vi "Start.vi"(8 "error in":errorcluster, 9 "timeout (-1)":i32=-1, 11 "Standard Engine Runtime in":refnum<class "Standard Engine Runtime.lvclass">) -> (0 "error out":errorcluster, 3 "Standard Engine Runtime out":refnum<class "Standard Engine Runtime.lvclass">)   [LabVIEW 2013, in "Standard Engine Runtime.lvclass"]
doc: "Sends a command for a paused but initialized engine to begin execution and enter the 'Running' state."
uses:
  Standard Engine Runtime.lvclass
  <vilib>/NI/Module Execution Interface/Engine Runtime/Execution States.ctl
  Standard Engine Runtime.lvclass/Standard Engine Runtime.ctl
  <vilib>/NI/Module Execution Interface/Engine Runtime/Engine Runtime Interface.lvclass
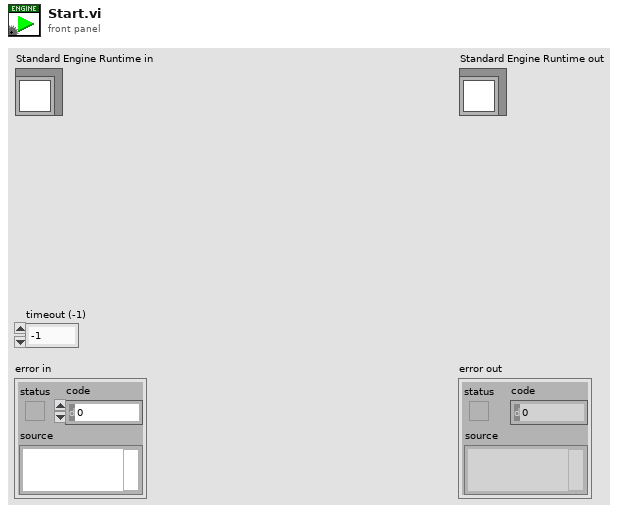
[diagram p1: front panel]
types:
  T1 = typedef "Engine Runtime Interface.lvclass/Execution States.ctl" = enum16{"Init", "Pre-Operational", "Safe-Operational", "Operational", "Stopped"}
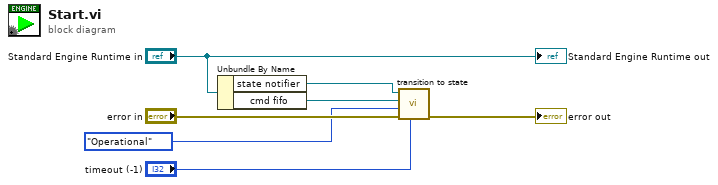
[diagram p0: block diagram]
diagram:
  n1 = Unbundle By Name("Standard Engine Runtime in") -> ("state notifier"=w3:refnum<notifier>, "cmd fifo"=w7:refnum<k33>)
  n2 = call "transition to state.vi"("timeout"="timeout (-1)", "error in"="error in", "States"=Execution_States."Operational" ("element"), "cmd fifo"=w7, "notifier"=w3) -> ("error out"=→"error out":errorcluster)  [unwired: 6 in]
  "Standard Engine Runtime out" <- "Standard Engine Runtime in"
